vi "Transmitter_no_IF.vi"() -> ()   [LabVIEW 2013]
uses:
  <vilib>/imath/engines/lvmath/Functions/Error Handling/error.ctl
  <vilib>/Analysis/2dsp.llb/Real FFT.vi
  <vilib>/imath/engines/lvmath2/RunTimeEngine/ErrorHandling/NIMS_Finalize Error.vi
  <vilib>/imath/engines/lvmath2/RunTimeEngine/Managers/WorkSpace/UID Generator.vi
  <vilib>/imath/engines/lvmath2/RunTimeEngine/NonStaticBuiltInFunctions/Manual/NIMS_NS_load.vi
  <vilib>/imath/engines/lvmath2/RunTimeEngine/RunTimeSymbolToken/NIMS_RunTimeSymbolToken_ResolveSymbol.vi
  <instcachedir>/0/NIMS_RunTimeSymbolToken_ResolveSymbol_F94DACEDB8D84373A3303A9E667D843C.lvgen/NIMS_RunTimeSymbolToken_ResolveSymbol_F94DACEDB8D84373A3303A9E667D843C_003.vi
  <vilib>/imath/engines/lvmath2/RunTimeEngine/Managers/SymbolTable/Write Variable.vi
  <vilib>/imath/engines/lvmath2/RunTimeEngine/LocalVariableDefStatement/MC_LocalVariableDefStatement_Display.vi
  <vilib>/imath/engines/lvmath2/RunTimeEngine/CommandStatement/NIMS_CommandStatement_MaskErr.vi
  <vilib>/imath/engines/lvmath2/RunTimeEngine/Managers/SymbolTable/Read Variable.vi
  <vilib>/imath/engines/lvmath2/RunTimeEngine/RunTimeType/NIMS_RunTimeType_Get Case Value.vi
  <vilib>/imath/engines/lvmath2/RunTimeEngine/NodeEndStatement/MC_NodeEndStatement_Dispose.vi
  <vilib>/imath/engines/lvmath2/RunTimeEngine/NodeEndStatement/NIMS_NodeEndStatement_Output.vi
  <instcachedir>/0/NIMS_NodeEndStatement_Output_53EC0D466D134D7ABD903AC30B43404B.lvgen/NIMS_NodeEndStatement_Output_53EC0D466D134D7ABD903AC30B43404B_016.vi
  <vilib>/imathl/engines/lvmath/Functions/Error Handling/Create Error.vi
  <vilib>/imath/engines/lvmath2/RunTimeEngine/RunTimeType/NIMS_RunTimeType_To Numeric.vi
  <instcachedir>/0/NIMS_RunTimeType_To Numeric_4795FB10E831402FABFA341B47E20681.lvgen/NIMS_RunTimeType_To Numeric_4795FB10E831402FABFA341B47E20681_000.vi
  <vilib>/imath/engines/lvmath2/RunTimeEngine/NodeEndStatement/NIMS_NodeEndStatement_Get Vector.vi
  <instcachedir>/0/NIMS_NodeEndStatement_Get Vector_BE4364D373AE46158CA0B14DEB6F98C8.lvgen/NIMS_NodeEndStatement_Get Vector_BE4364D373AE46158CA0B14DEB6F98C8_003.vi
  <vilib>/imath/engines/lvmath/Plug In/_Char/RunTimeType/NIMS_CH_RunTimeType_To Character 2D.vi
  <instcachedir>/0/NIMS_NodeEndStatement_Get Vector_BE4364D373AE46158CA0B14DEB6F98C8.lvgen/NIMS_NodeEndStatement_Get Vector_BE4364D373AE46158CA0B14DEB6F98C8_000.vi
  <vilib>/imath/engines/lvmath/Plug In/_Char/NIMS_CH_Character 1D to U8 1D.vi
  <vilib>/imath/engines/lvmath2/RunTimeEngine/BuiltInFunctions/length/NIMS_length(GV).vi
  <instcachedir>/0/NIMS_length(GV)_08A3D13377FD4E4B96F5795FBF3698FA.lvgen/NIMS_length(GV)_08A3D13377FD4E4B96F5795FBF3698FA_004.vi
  <vilib>/imath/engines/lvmath2/RunTimeEngine/BuiltInFunctions/zeros/NIMS_V=zeros(I32,I32).vi
  <vilib>/imath/engines/lvmath2/RunTimeEngine/Managers/SymbolTable/Clear UID.vi
  <instcachedir>/0/NIMS_NodeEndStatement_Output_53EC0D466D134D7ABD903AC30B43404B.lvgen/NIMS_NodeEndStatement_Output_53EC0D466D134D7ABD903AC30B43404B_011.vi
  <vilib>/imath/engines/lvmath2/RunTimeEngine/IndexRead/NIMS V(R3).vi
  <instcachedir>/0/NIMS V(R3)_BB7B7B2F47B844E7B6C44853B6A6C035.lvgen/NIMS V(R3)_BB7B7B2F47B844E7B6C44853B6A6C035_000.vi
  <vilib>/imath/engines/lvmath2/RunTimeEngine/IndexReplace/NIMS V(R3)=V.vi
  <instcachedir>/0/NIMS V(R3)=V_69F337331DAD430986A98313EEA6EC3D.lvgen/NIMS V(R3)=V_69F337331DAD430986A98313EEA6EC3D_000.vi
  <vilib>/imath/engines/lvmath2/RunTimeEngine/RunTimeType/NIMS_RunTimeType_From StrictType (excl LVString).vi
  <instcachedir>/0/NIMS_RunTimeType_From StrictType (excl LVString)_4DEE718D6EB74582AA20236969C084FC.lvgen/NIMS_RunTimeType_From StrictType (excl LVString)_4DEE718D6EB74582AA20236969C084FC_000.vi
  <vilib>/imath/engines/lvmath2/RunTimeEngine/ErrorHandling/NIMS_Create Error From Enums.vi
  <vilib>/imath/engines/lvmath2/RunTimeEngine/BuiltInFunctions/repeatmx/NIMS_repeatmx(GM, I32, I32).vi
  <instcachedir>/0/NIMS_repeatmx(GM, I32, I32)_71D32CAC8D434697AB9DA7B55FCB46E4.lvgen/NIMS_repeatmx(GM, I32, I32)_71D32CAC8D434697AB9DA7B55FCB46E4_004.vi
  <instcachedir>/0/NIMS_length(GV)_08A3D13377FD4E4B96F5795FBF3698FA.lvgen/NIMS_length(GV)_08A3D13377FD4E4B96F5795FBF3698FA_003.vi
  <vilib>/imath/engines/lvmath2/RunTimeEngine/RowToken/NIMS_RowToken_M_SorRV.vi
  <instcachedir>/0/NIMS_RowToken_M_SorRV_6464340A296F47B6970F468C8541F43A.lvgen/NIMS_RowToken_M_SorRV_6464340A296F47B6970F468C8541F43A_004.vi
  <instcachedir>/0/NIMS_NodeEndStatement_Output_53EC0D466D134D7ABD903AC30B43404B.lvgen/NIMS_NodeEndStatement_Output_53EC0D466D134D7ABD903AC30B43404B_005.vi
  <vilib>/imath/engines/lvmath2/RunTimeEngine/RangeToken/NIMS_Range.vi
  <instcachedir>/0/NIMS_Range_7481B155BEE341ECA0F59DDB444E2C09.lvgen/NIMS_Range_7481B155BEE341ECA0F59DDB444E2C09_000.vi
  <vilib>/imath/engines/lvmath2/RunTimeEngine/IndexRead/NIMS V(R2).vi
  <instcachedir>/0/NIMS V(R2)_C76619605A0E4E9F8B2FA9389712AC47.lvgen/NIMS V(R2)_C76619605A0E4E9F8B2FA9389712AC47_000.vi
  <vilib>/imath/engines/lvmath2/RunTimeEngine/BuiltInFunctions/mirrorh/NIMS_mirrorh(GRowV).vi
  <instcachedir>/0/NIMS_mirrorh(GRowV)_B6A8CC4EAFBA4F9A82A59460D67BDFF0.lvgen/NIMS_mirrorh(GRowV)_B6A8CC4EAFBA4F9A82A59460D67BDFF0_000.vi
  LabVIEW Data/MathScriptVIs/MCStatic_31879994332_3c241b7dddb4c004da928be36820582d.vi
  <instcachedir>/0/MCStatic_31879994332_3c241b7dddb4c004da928be36820582d_29D772E1BAF74A5FB4AED162C6C5D09D.lvgen/MCStatic_31879994332_3c241b7dddb4c004da928be36820582d_29D772E1BAF74A5FB4AED162C6C5D09D_000.vi
  <instcachedir>/0/NIMS_NodeEndStatement_Output_53EC0D466D134D7ABD903AC30B43404B.lvgen/NIMS_NodeEndStatement_Output_53EC0D466D134D7ABD903AC30B43404B_000.vi
  LabVIEW Data/MathScriptVIs/MCStatic_31879994332_c19998dbed1c0366eafca5becc38f78d.vi
  <instcachedir>/0/MCStatic_31879994332_c19998dbed1c0366eafca5becc38f78d_8EA7CB7CD67A4BF8AAB5A0C0F881FA84.lvgen/MCStatic_31879994332_c19998dbed1c0366eafca5becc38f78d_8EA7CB7CD67A4BF8AAB5A0C0F881FA84_002.vi
  <vilib>/imath/engines/lvmath2/RunTimeEngine/BuiltInFunctions/numelements/NIMS_numelements.vi
  <instcachedir>/0/NIMS_numelements_A776DA77F73142F68C2F209B523114C5.lvgen/NIMS_numelements_A776DA77F73142F68C2F209B523114C5_003.vi
  <vilib>/imath/engines/lvmath2/RunTimeEngine/BuiltInFunctions/close/NIMS_close(Enums).vi
  <instcachedir>/0/NIMS V(R2)_C76619605A0E4E9F8B2FA9389712AC47.lvgen/NIMS V(R2)_C76619605A0E4E9F8B2FA9389712AC47_001.vi
  <vilib>/imath/engines/lvmath2/RunTimeEngine/BuiltInFunctions/abs/NIMS_abs(signed).vi
  <instcachedir>/0/NIMS_abs(signed)_C4FCB8E6058B49B797C7C8D53CA5F6EC.lvgen/NIMS_abs(signed)_C4FCB8E6058B49B797C7C8D53CA5F6EC_006.vi
  <vilib>/imath/engines/lvmath2/RunTimeEngine/BuiltInFunctions/max/1 input/NIMS_max(RV).vi
  <instcachedir>/0/NIMS_max(RV)_237633DB1D604D5BA7001287DF3C7957.lvgen/NIMS_max(RV)_237633DB1D604D5BA7001287DF3C7957_000.vi
  <instrlib>/niUSRP/niUSRP Write Tx Data (CDB Cluster).vi
  MATLAB_func/rtrcpulse.m
  MATLAB_func/TX_RRC_filtering.m
  <vilib>/imath/engines/lvmath2/RunTimeEngine/Managers/SymbolTable/NIMS_WorkSpace.lvlib
  <vilib>/Analysis/NI_AALPro.lvlib
panel:
  out "total number of bits":i32
  out "Waveform Graph 6":dbl[](graph)
  in  "loop control":bool
  out "coerced carrier frequency":dbl=100000.0 format="%#_6p"
  in  "stop":bool
  in  "file (use dialog)":path=path "C:/Users/Lab/Downloads/FPGA.JPG"
  out "number of data bits":i32
  out "x/y":fxp<+,27,27>
  out "a":cdb[](array[numeric])
  out "L":i32
  out "wave":cdb[](array[numeric])
  in  "number of bits (per block)":dbl
  in  "channel list":string
  out "coerced gain":dbl format="%#_6f"
  out "coerced IQ rate":dbl=100000.0 format="%#_6p"
  in  "active antenna":string
  in  "gain":dbl format="%#_6f"
  in  "IQ rate":dbl=1000000.0 format="%#_6p"
  # "continous"
  # "single shot"
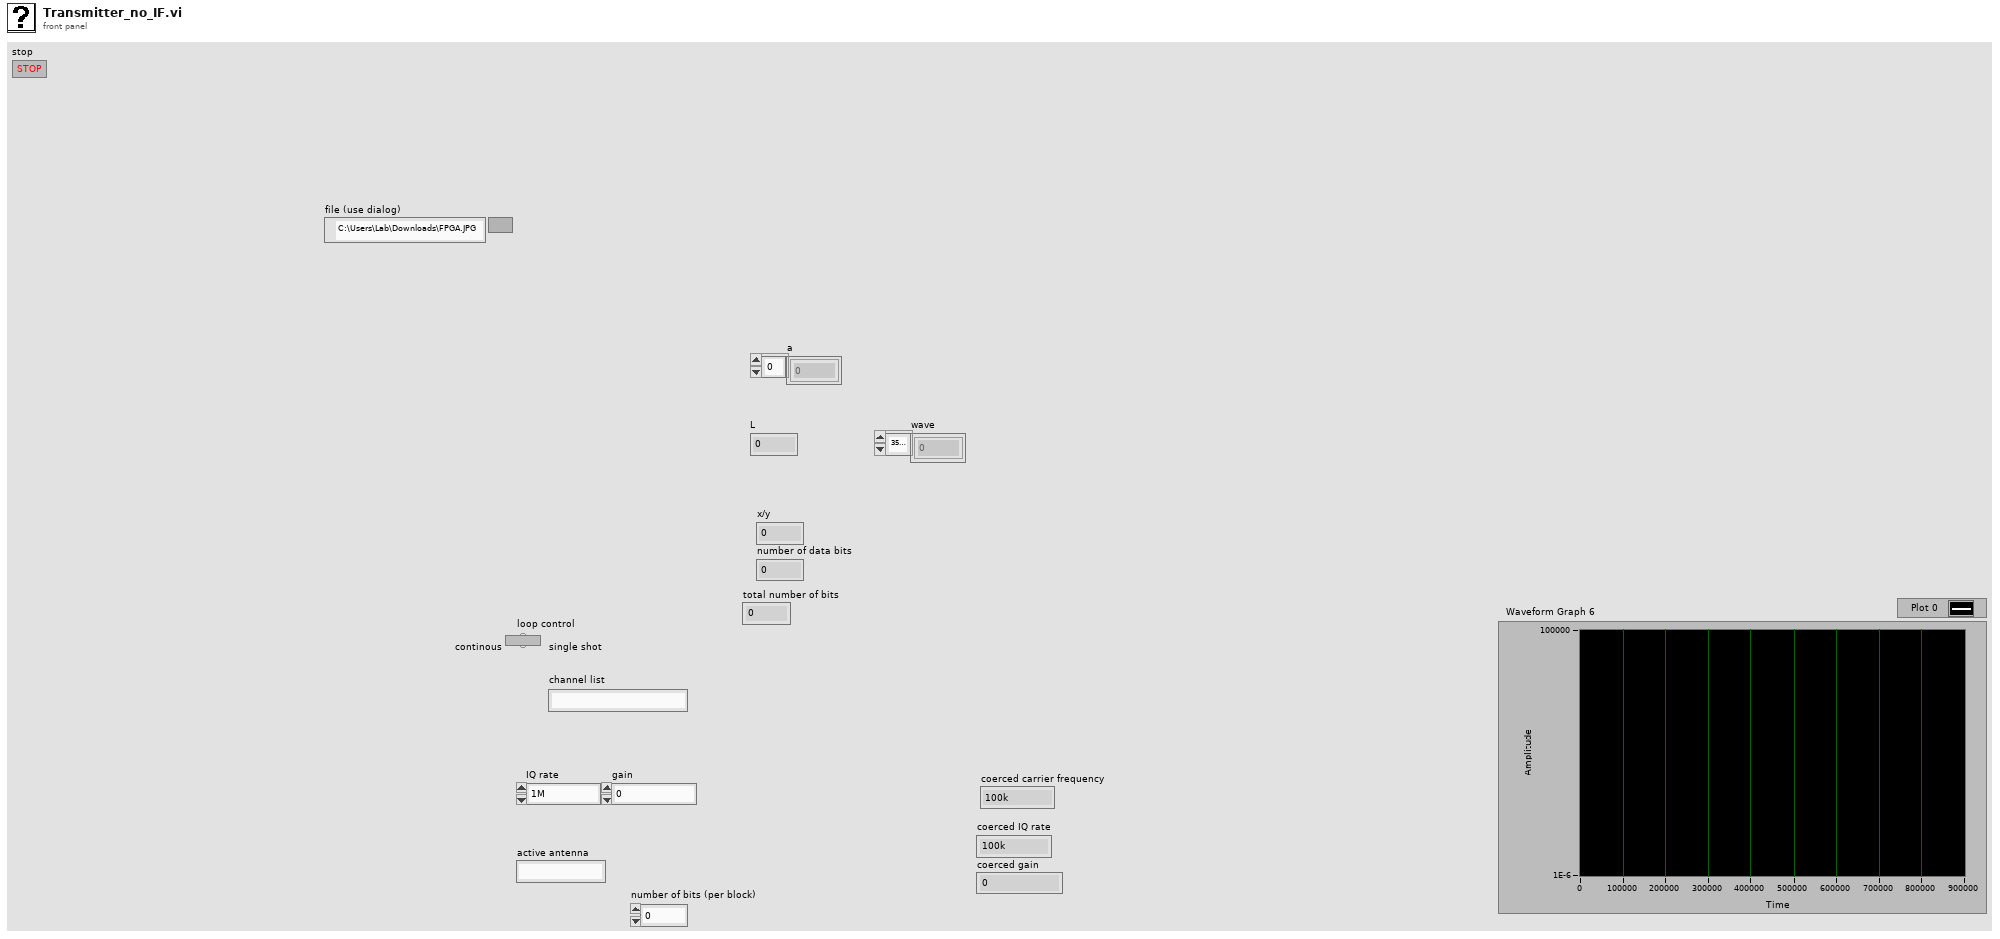
[diagram p1: front panel]
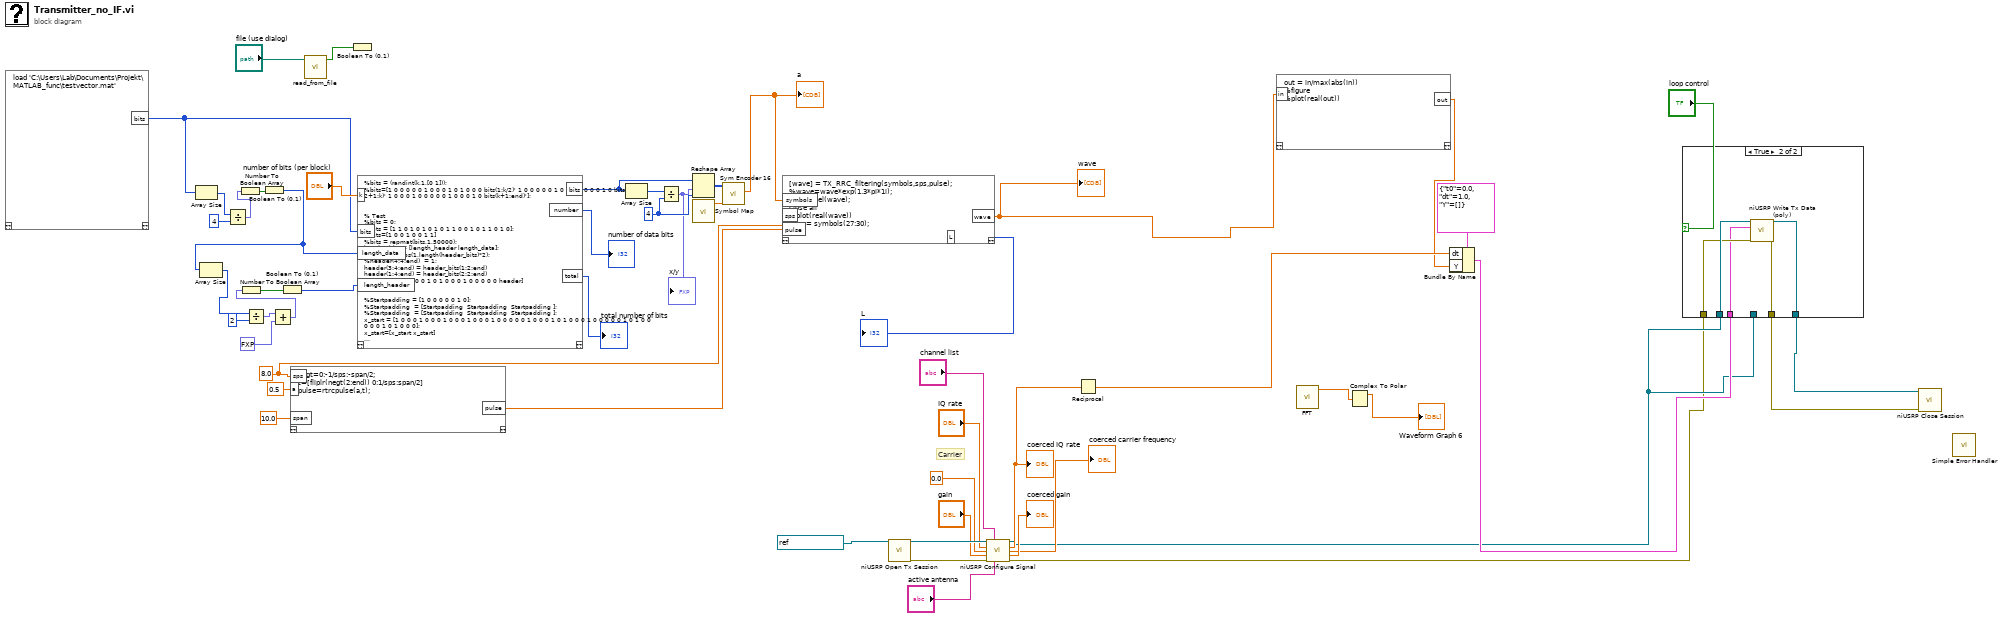
[diagram p0: block diagram]
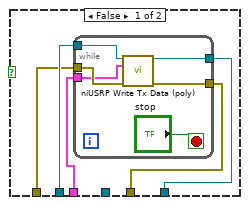
[diagram p2: hidden frame]
diagram:
  w34 = 8.0 ("sps")
  w42 = 4 ("dimension size")
  # "Carrier"
  n1 = mathscript code="load 'C:\\Users\\Lab\\Documents\\Projekt\\MATLAB_func\\testvector.mat'"() -> ("bits"=w15:u32[])  [unwired: 1 in, 1 out]
  n2 = Array Size(array=w15) -> (size(s)=w32:i32)
  n3 = Divide(x=w32, y=4) -> (x/y=w31:fxp<+,32,32>)
  n4 = Number To Boolean Array(number=w31) -> (Boolean array=w33:bool[])
  n5 = Boolean To (0,1)(Boolean=w33) -> (0, 1=w7:i16[])
  n6 = Array Size(array=w7) -> (size(s)=w6:i32)
  n7 = Divide(x=w6, y=2) -> (x/y=w27:fxp<+,9,9>)
  n8 = Add(x=w27, y=fxp<+,9,9> 5.0) -> (x+y=w24:fxp<+,10,10>)
  n9 = Number To Boolean Array(number=w24) -> (Boolean array=w29:bool[])
  n10 = Boolean To (0,1)(Boolean=w29) -> (0, 1=w26:i16[])
  n11 = mathscript code="negt=0:-1/sps:-span/2;\nt=[fliplr(negt(2:end)) 0:1/sps:span/2]\npulse=rtrcpulse(a,t);"("sps"=w34, "span"=10.0, "a"=0.5) -> ("pulse"=w35:dbl[])  [unwired: 1 in, 1 out]
  n12 = call "read_from_file.vi"("file (use dialog)"="file (use dialog)") -> ("data"=w16:bool[])  [unwired: 10 in]
  n13 = Boolean To (0,1)(Boolean=w16) -> ()  [unwired: 1 out]
  n14 = mathscript code="%bits = (randint(k,1,[0 1]));\n%bits=[1 0 0 0 0 0 1 0 0 0 1 0 1 0 0 0 bits(1:k/2)' 1 0 0 0 0 0 1 0 1 0 0 0 0 0 1 0 bits(k/2+1:k)' 1 0 0 0 1 0 0 0 0 0 1 0 0 0 1 0 bits(k+1:end)'];\n\n\n% Test\n%bits = 0;\n%bits = [1 1 0 1 0 1 0 1 0 1 1 0 0 1 0 1 1 0 1 0];\n%bits=[1 0 0 1 0 0 1 1]\n%bits = repmat(bits,1,50000);\nheader_bits = [length_header length_data];\nheader = zeros(1,length(header_bits)*2);\n%header(4:4:end)  = 1;\nheader(3:4:end) = header_bits(1:2:end)\nheader(1:4:end) = header_bits(2:2:end)\n%header = [1 0 0 0 1 0 1 0 0 0 1 0 0 0 0 0 header]\n\n\n%Startpadding = [1 0 0 0 0 0 1 0];\n%Startpadding  = [Startpadding  Startpadding  Startpadding ];\n%Startpadding  = [Startpadding  Startpadding  Startpadding ];\nx_start = [1 0 0 0 1 0 0 0 1 0 0 0 1 0 0 0 1 0 0 0 0 0 1 0 0 0 1 0 1 0 0 0 1 0 0 0 0 0 1 0 1 0 0 0 0 0 1 0 1 0 0 0];\nx_start=[x_start x_start]\n\n% Test of 11 bits Barker sequence.\n% x_start = [1 0 0 0 1 0 0 0 1 0 0 0 0 0 1 0 0 0 1 0 0 0 1 0 1 0 0 0 0 0 1 0 0 0 1 0 1 0 0 0 0 0 1 0]\n\n%test_start = [0 1 0 1 1 1 0 0 1 0 1 1 0 1 0 0 0 0 1 0 1 1 1 0 1 1 0 1 0 0 0 0 0 1 1 1 0 0 0 1 1 0 0 0 1 0 1 0 0 0 1 1 1 1 1 1 0 1 1 0 1 0 0 1];\n%test_start = randint(1,65536,[0 1]);\n%test_start=[0 0 0 0 1 0 1 0 0 1 0 1 1 1 1 1 0 0 0 0 1 0 1 0]\ntest_start=[0 0 0 0 1 0 1 0]\ntest_start = repmat(test_start,1,3200)\n\n%bits=[1 0 0 1 0 0 1 1]\n%bits = repmat(bits,1,1600)\n%test_start = repmat(test_start,1,500);\n\n%bits = [0 1 0 1 1 1 0 1 0 0 1 0 0 1 0 1 1 1 1 0 0 1 0 1 0 0 0 1 1 1 0 0 1 0 1 0 1 0 1 0 1 bits];\n\n% bits = [randint(1,4096,[0 1]) test_start x_start bits];\nnumber=length(bits);\nbits = [test_start x_start bits];\ntotal=length(bits)"("k"="number of bits (per block)", "bits"=w15, "length_data"=w7, "length_header"=w26) -> ("bits"=w39:u32[], "number"=→"number of data bits":i32, "total"=→"total number of bits":i32)  [unwired: 1 in, 1 out]
  n15 = Array Size(array=w39) -> (size(s)=w40:i32)
  n16 = Divide(x=w40, y=w42) -> (x/y=w41:fxp<+,27,27>)
  "x/y" <- w41
  n17 = Reshape Array(w39, w41, w42) -> (w43:u32[][])
  n18 = call "Symbol Map.vi"() -> ("symbol_map"=w44:cdb[])  [unwired: 11 in]
  n19 = call "Sym Encoder 16.vi"("symbol_map"=w44, "b"=w43) -> ("a"=w38:cdb[])  [unwired: 9 in]
  "a" <- w38
  n20 = mathscript code="[wave] = TX_RRC_filtering(symbols,sps,pulse);\n%wave=wave*exp(1.3*pi*1i);\nL = numel(wave);\nclose all\n%plot(real(wave))\nsym = symbols(27:30);"("symbols"=w38, "pulse"=w35, "sps"=w34) -> ("wave"=w14:cdb[], "L"=→"L":i32)  [unwired: 1 in, 1 out]
  "wave" <- w14
  n21 = call <instrlib>:"niUSRP Open Tx Session.vi"("device names"=refnum<k15> "192.168.10.8") -> ("session handle out"=w53:refnum<k15>, "error out"=w52:errorcluster)  [unwired: 13 in]
  n22 = call <instrlib>:"niUSRP Configure Signal.vi"("session handle"=w53, "channel list"="channel list", "IQ rate"="IQ rate", "carrier frequency"=0.0, "gain"="gain", "error in (no error)"=w52, "active antenna"="active antenna") -> ("session handle out"=w11:refnum<k15>, "coerced IQ rate"=w18:dbl, "coerced carrier frequency"=→"coerced carrier frequency":dbl, "coerced gain"=→"coerced gain":dbl, "error out"=w8:errorcluster)  [unwired: 4 in]
  "coerced IQ rate" <- w18
  n23 = Reciprocal(x=w18) -> (1/x=w19:dbl)
  n24 = mathscript code="out = in/max(abs(in))\n%figure\n%plot(real(out))"("in"=w14) -> ("out"=w1:cdb[])  [unwired: 1 in, 1 out]
  n25 = call-poly <vilib>:"FFT.vi"() -> ("FFT {X}"=w4:cdb[])  [unwired: 10 in, 1 out]
  n26 = Complex To Polar(r * e^(i*theta)=w4) -> (r=→"Waveform Graph 6":dbl[])  [unwired: 1 out]
  n27 = Bundle By Name(cluster=cluster{"t0":dbl, "dt":dbl, "Y":cdb[]} {"t0"=0.0, "dt"=1.0, "Y"=[]} ("data"), "dt"=w19, "Y"=w1) -> (w12:cluster{"t0":dbl, "dt":dbl, "Y":cdb[]})
  n28 = case shown="True" "loop control" {
    tunnel: w11 -> [w58 w69]
    tunnel: w12 -> [w54 w65]
    tunnel: w11 -> [_ _]
    tunnel: [w55 w68] -> w10
    tunnel: [w56 w67] -> w9
    tunnel: w8 -> [w57 w66]
    frame False {
      n29 = while {
        tunnel: w57 -> [w62]
        tunnel: w58 -> [w63]
        tunnel: [w61] -> w56
        tunnel: [w60] -> w55
        tunnel: w54 -> [w59]
        stop <- "stop" stop-if-true
        n30 = call-poly <instrlib>:"niUSRP Write Tx Data (poly).vi"("session handle"=w63, "data"=w59, "error in (no error)"=w62) -> ("session handle out"=w61:refnum<k15>, "error out"=w60:errorcluster)  [unwired: 11 in]
      }
    }
    frame True {
      n31 = call-poly <instrlib>:"niUSRP Write Tx Data (poly).vi"("session handle"=w69, "data"=w65, "error in (no error)"=w66) -> ("session handle out"=w67:refnum<k15>, "error out"=w68:errorcluster)  [unwired: 11 in]
    }
  }
  n32 = call <instrlib>:"niUSRP Close Session.vi"("session handle"=w9, "error in (no error)"=w10) -> ()  [unwired: 13 in, 1 out]
  n33 = call <vilib>:"Simple Error Handler.vi"() -> ()  [unwired: 5 in, 5 out]
